vi "Agilent VNA Get Stimulus.vi"(7 "Agilent VNA":T1, 8 "error in (no error)":errorcluster, 9 "Channel":i8=1 min=1 max=99 step=1, 11 "VISA Resource Name":refnum<visa-resource-name>) -> (0 "error out":errorcluster, 2 "SP Stimulus":T2={"Use Instrument Settings"=FALSE, "Blank Frequencies"=FALSE, "Sweep Type"=enum."Linear", "Sweep"={"Fstart"=500.0, "Fstop"=1500.0, "Units"=enum."MHz", "Points"=201}, "Power (dBm)"=999.0, "IFBW (Hz)"=-1.0, "Sweep Time (s)"=-1.0, "Calibration"={"State"=FALSE, "String"=""}} {"Sweep Time (s)" format="%.3g"}, 3 "dup VISA Resource Name":refnum<visa-resource-name>)   [LabVIEW 2011]
uses:
  tests/S Parameter/TypeDefs/SP Stimulus Parameters.ctl
  tests/S Parameter/TypeDefs/SP Frequency Units.ctl
  tests/S Parameter/TypeDefs/SP Calibration State.ctl
  TypeDefs/Agilent VNA Instrument Info.ctl
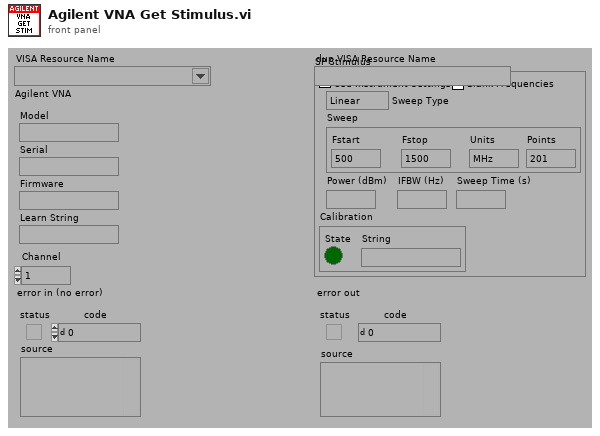
[diagram p1: front panel]
types:
  T1 = typedef "Agilent VNA Instrument Info.ctl" = cluster{"Model":string, "Serial":string, "Firmware":string, "Learn String":string}
  T2 = typedef "SP Stimulus Parameters.ctl" = cluster{"Use Instrument Settings":bool, "Blank Frequencies":bool, "Sweep Type":enum32{"Linear", "Logarithmic", "List", "Power", "CW"}, "Sweep":cluster{"Fstart":dbl, "Fstop":dbl, "Units":T3, "Points":i32}, "Power (dBm)":dbl, "IFBW (Hz)":dbl, "Sweep Time (s)":dbl, "Calibration":T4}
  T3 = typedef "SP Frequency Units.ctl" = enum16{"Hz", "kHz", "MHz", "GHz", "Points"}
  T4 = typedef "SP Calibration State.ctl" = cluster{"State":bool, "String":string}
  T5 = typedef "Agilent VNA Sweep Type.ctl" = enum32{"Linear Sweep", "Logarithmic Sweep", "Frequency List", "CW Time Sweep", "Power Sweep"}
  T6 = enum32{"Linear", "Logarithmic", "List", "Power", "CW"}
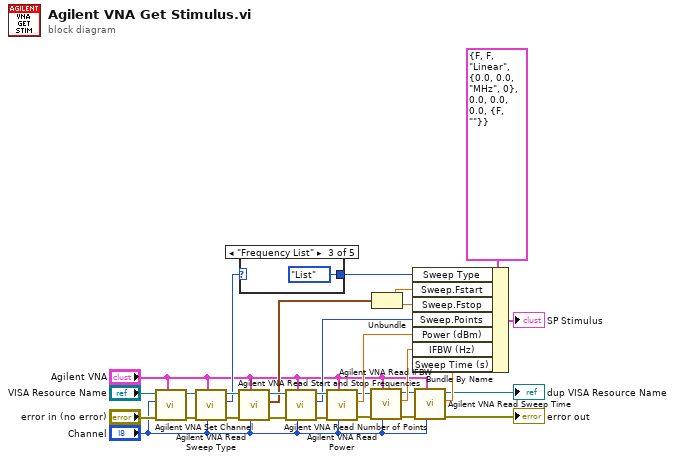
[diagram p0: block diagram]
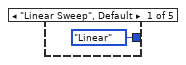
[diagram p2: hidden frame]
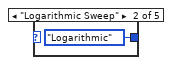
[diagram p3: hidden frame]
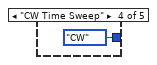
[diagram p4: hidden frame]
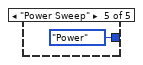
[diagram p5: hidden frame]
diagram:
  n1 = call "Agilent VNA Set Channel.vi"("Agilent VNA"="Agilent VNA", "error in (no error)"="error in (no error)", "Channel"="Channel", "VISA Resource Name"="VISA Resource Name") -> ("error out"=w3:errorcluster, "dup VISA Resource Name"=w4:refnum<visa-resource-name>)  [unwired: 6 out]
  n2 = call "Agilent VNA Read Sweep Type.vi"("Channel"="Channel", "Agilent VNA"="Agilent VNA", "error in (no error)"=w3, "VISA Resource Name"=w4) -> ("error out"=w26:errorcluster, "Sweep Type"=w12:T5, "dup VISA Resource Name"=w25:refnum<visa-resource-name>)  [unwired: 5 out]
  n3 = call "Agilent VNA Read Start and Stop Frequencies.vi"("Channel"="Channel", "Agilent VNA"="Agilent VNA", "error in (no error)"=w26, "VISA Resource Name"=w25) -> ("error out"=w24:errorcluster, "Start/Stop Freqs, MHz"=w8:cluster{"Fstart":dbl, "Fstop":dbl}, "dup VISA Resource Name"=w23:refnum<visa-resource-name>)  [unwired: 5 out]
  n4 = case shown="\"Frequency List\"" w12 {
    tunnel: [T6."Linear" ("Sweep Type") T6."Logarithmic" ("Sweep Type") T6."List" ("Sweep Type") T6."CW" ("Sweep Type") T6."Power" ("Sweep Type")] -> w7
    frame "Linear Sweep", Default {
    }
    frame "Logarithmic Sweep" {
    }
    frame "Frequency List" {
    }
    frame "CW Time Sweep" {
    }
    frame "Power Sweep" {
    }
  }
  n5 = call "Agilent VNA Read Number of Points.vi"("Channel"="Channel", "Agilent VNA"="Agilent VNA", "error in (no error)"=w24, "VISA Resource Name"=w23) -> ("error out"=w19:errorcluster, "Number Points"=w11:i32, "dup VISA Resource Name"=w20:refnum<visa-resource-name>)  [unwired: 5 out]
  n6 = call "Agilent VNA Read Power.vi"("Channel"="Channel", "Agilent VNA"="Agilent VNA", "error in (no error)"=w19, "VISA Resource Name"=w20) -> ("error out"=w21:errorcluster, "Source Power, dBm"=w27:dbl, "dup VISA Resource Name"=w22:refnum<visa-resource-name>)  [unwired: 5 out]
  n7 = call "Agilent VNA Read IFBW.vi"("Channel"="Channel", "Agilent VNA"="Agilent VNA", "error in (no error)"=w21, "VISA Resource Name"=w22) -> ("error out"=w17:errorcluster, "IFBW, Hz"=w28:dbl, "dup VISA Resource Name"=w18:refnum<visa-resource-name>)  [unwired: 5 out]
  n8 = Unbundle(w8) -> ("Fstart"=w10:dbl, "Fstop"=w9:dbl)
  n9 = call "Agilent VNA Read Sweep Time.vi"("Channel"="Channel", "Agilent VNA"="Agilent VNA", "error in (no error)"=w17, "VISA Resource Name"=w18) -> ("error out"=→"error out":errorcluster, "Sweep Time, s"=w16:dbl, "dup VISA Resource Name"=→"dup VISA Resource Name":refnum<visa-resource-name>)  [unwired: 5 out]
  n10 = Bundle By Name(cluster=T2 {"Use Instrument Settings"=FALSE, "Blank Frequencies"=FALSE, "Sweep Type"=enum."Linear", "Sweep"={"Fstart"=0.0, "Fstop"=0.0, "Units"=enum."MHz", "Points"=0}, "Power (dBm)"=0.0, "IFBW (Hz)"=0.0, "Sweep Time (s)"=0.0, "Calibration"={"State"=FALSE, "String"=""}} ("Stimulus"), "Sweep Type"=w7, "Sweep.Fstart"=w10, "Sweep.Fstop"=w9, "Sweep.Points"=w11, "Power (dBm)"=w27, "IFBW (Hz)"=w28, "Sweep Time (s)"=w16) -> (→"SP Stimulus":T2)
